vi "CalcRmr0Kappa.vi"(0 "dvotAFTKinetics":refnum<class "dvotAFTKinetics.lvclass">, 1 "kParNum":i32, 2 "kParVal":dbl, 3 "annealingModel":i32, 4 "rmr0":dbl, 5 "error in (no error)":errorcluster, 7 "kappa":dbl) -> (14 "dvotAFTKinetics":refnum<class "dvotAFTKinetics.lvclass">, 15 "rmr0 out":dbl, 16 "kappa out":dbl, 19 "error out":errorcluster)   [LabVIEW 2012, in "dvotAFTKinetics.lvclass"]
uses:
  dvotAFTKinetics.lvclass
  Constants/dvotAFTConstants.vi
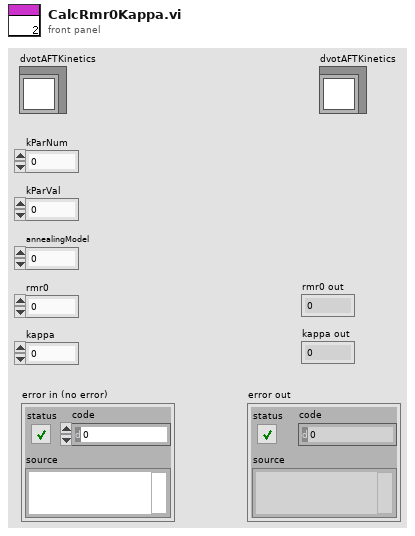
[diagram p1: front panel]
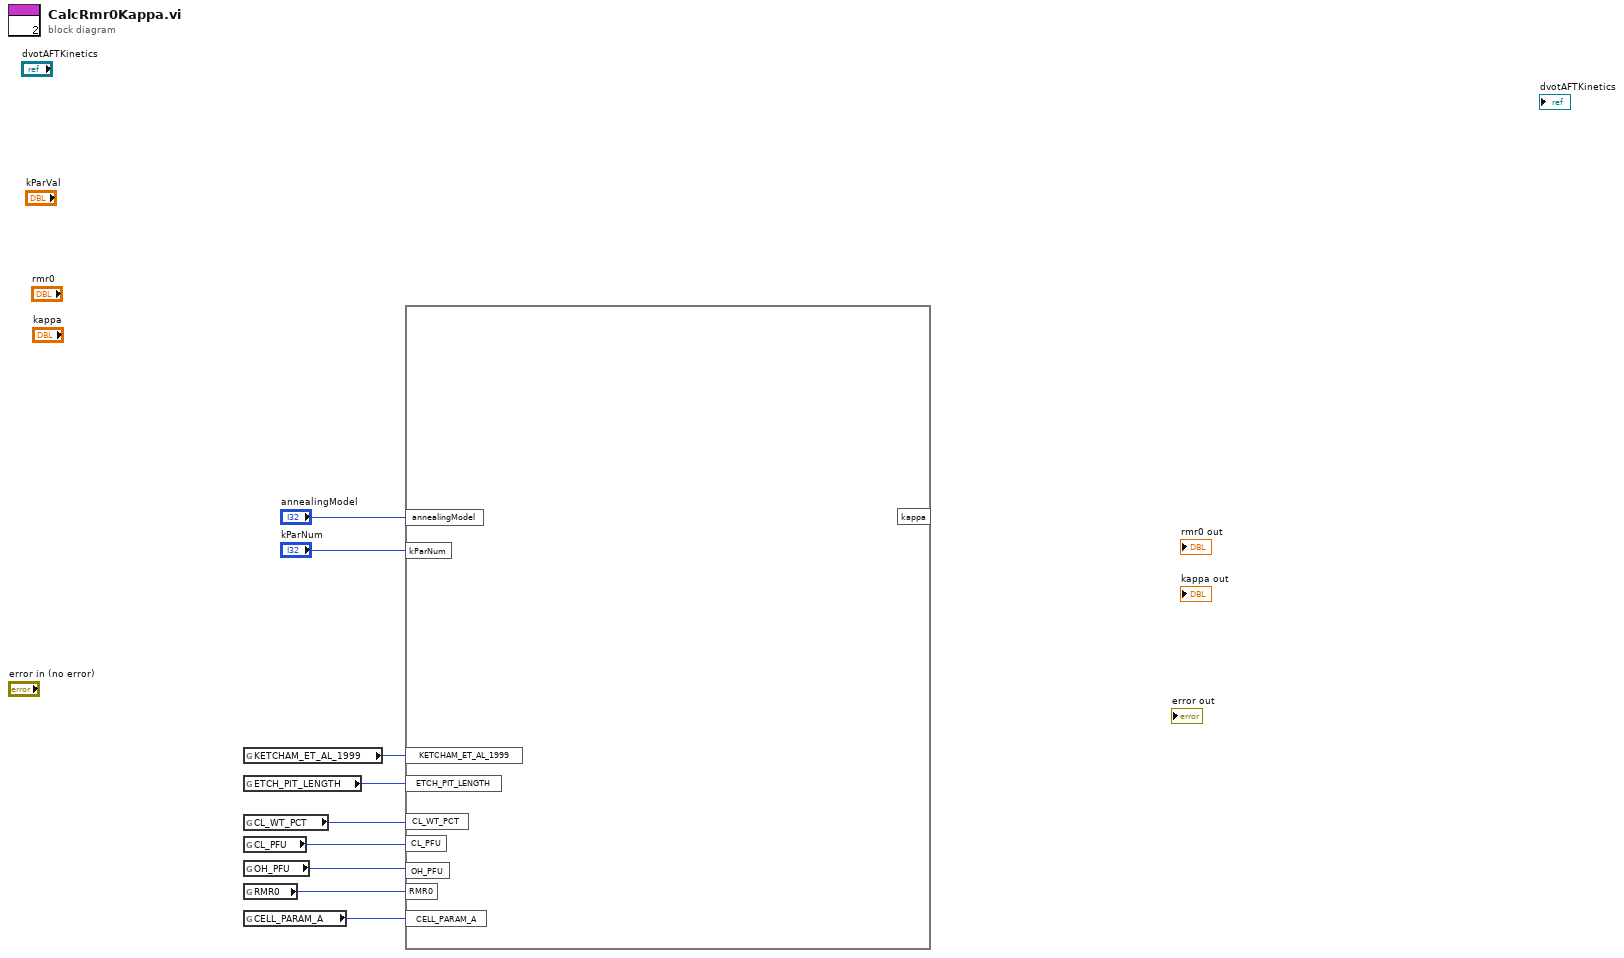
[diagram p0: block diagram]
diagram:
  n1 = global read "dvotAFTConstants.vi" "KETCHAM_ET_AL_1999"() -> (w8:i32)
  n2 = global read "dvotAFTConstants.vi" "ETCH_PIT_LENGTH"() -> (w7:i32)
  n3 = global read "dvotAFTConstants.vi" "CL_WT_PCT"() -> (w2:i32)
  n4 = global read "dvotAFTConstants.vi" "CL_PFU"() -> (w1:i32)
  n5 = global read "dvotAFTConstants.vi" "OH_PFU"() -> (w3:i32)
  n6 = global read "dvotAFTConstants.vi" "RMR0"() -> (w4:i32)
  n7 = global read "dvotAFTConstants.vi" "CELL_PARAM_A"() -> (w5:i32)
  n8 = formula code=""("annealingModel"="annealingModel", "KETCHAM_ET_AL_1999"=w8, "ETCH_PIT_LENGTH"=w7, "kParNum"="kParNum", "CL_WT_PCT"=w2, "CL_PFU"=w1, "OH_PFU"=w3, "RMR0"=w4, "CELL_PARAM_A"=w5) -> ()  [unwired: 1 out]
